vi "F2ToFalseColor.vi"(1 "Intensity":u32[][][][](array[numeric]), 2 "Plane":u32, 3 "Threshold (max)":cluster{"max":u32, "min":u32}) -> (0 "FalseColor":u32[][](array[numeric]))   [LabVIEW 2009]
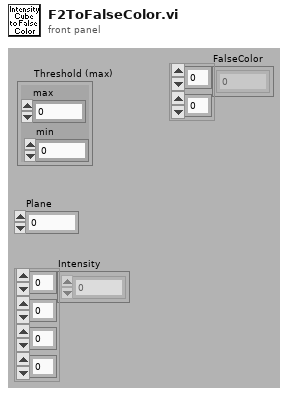
[diagram p1: front panel]
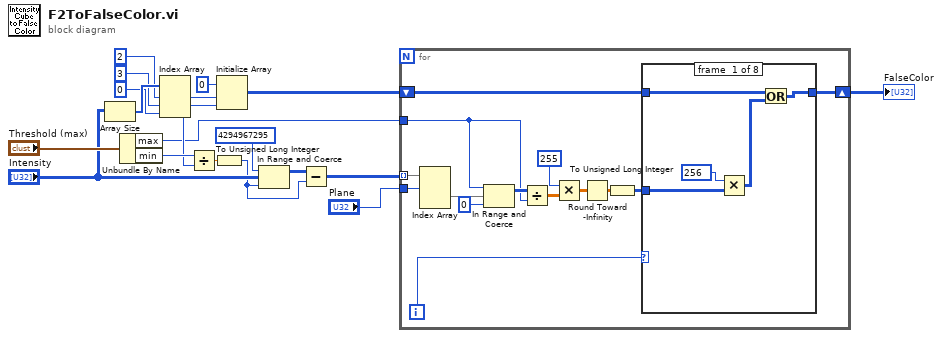
[diagram p0: block diagram]
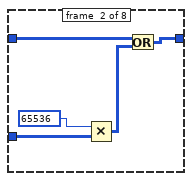
[diagram p2: hidden frame]
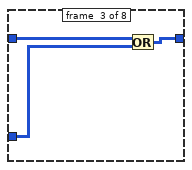
[diagram p3: hidden frame]
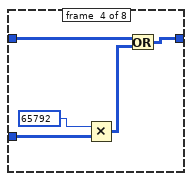
[diagram p4: hidden frame]
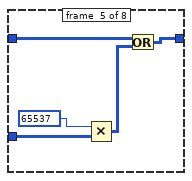
[diagram p5: hidden frame]
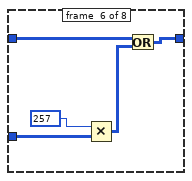
[diagram p6: hidden frame]
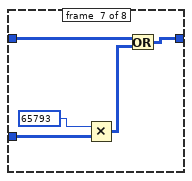
[diagram p7: hidden frame]
diagram:
  n1 = Array Size(array="Intensity") -> (size(s)=w17:i32[])
  n2 = Unbundle By Name("Threshold (max)") -> ("max"=w1:u32, "min"=w9:u32)
  n3 = Index Array(array=w17, index #1=2 ("index"), index #2=3 ("index"), index #3=0 ("index")) -> (element #1=w11:i32, element #2=w10:i32, element #3=w8:i32)
  n4 = Divide(x=w9, y=w8) -> (x/y=w7:dbl)
  n5 = To Unsigned Long Integer(number=w7) -> (unsigned 32bit integer=w4:u32)
  n6 = Initialize Array(u32 0, w11, w10) -> (w14:u32[][])
  n7 = In Range and Coerce(upper limit=u32 4294967295 ("index"), x="Intensity", lower limit=w4) -> (coerced(x)=w5:u32[][][][])  [unwired: 1 out]
  n8 = Subtract(x=w5, y=w4) -> (x-y=w2:u32[][][][])
  n9 = for {
    tunnel: w2 -> [w34] mode=indexing
    tunnel: "Plane" -> [w33]
    shift-right: [w22] -> w20
    shift-left: w14 -> [w23]
    tunnel: w1 -> [w21]
    i -> [w30]
    n10 = Index Array(array=w34, index (dim 0)=w33) -> (element=w32:u32[][])  [unwired: 2 in]
    n11 = In Range and Coerce(upper limit=w21, x=w32, lower limit=u32 0) -> (coerced(x)=w29:u32[][])  [unwired: 1 out]
    n12 = Divide(x=w29, y=w21) -> (x/y=w28:dbl[][])
    n13 = Multiply(x=u32 255 ("Threshold (max)"), y=w28) -> (x*y=w26:dbl[][])
    n14 = Round Toward -Infinity(1:w26) -> (0:w25:dbl[][])
    n15 = To Unsigned Long Integer(number=w25) -> (unsigned 32bit integer=w24:u32[][])
    n16 = case shown="3" w30 {
      tunnel: w24 -> [w39 w44 w45 w52 w57 w62 w67 _]
      tunnel: w23 -> [w36 w41 w47 w49 w54 w59 w64 w68]
      tunnel: [w35 w40 w46 w48 w53 w58 w63 w68] -> w22
      frame #0 {
        n17 = Multiply(x=u32 256 ("Threshold (max)"), y=w39) -> (x*y=w37:u32[][])
        n18 = Or(x=w36, y=w37) -> (x .or. y?=w35:u32[][])
      }
      frame #1 {
        n19 = Multiply(x=u32 65536 ("Threshold (max)"), y=w44) -> (x*y=w42:u32[][])
        n20 = Or(x=w41, y=w42) -> (x .or. y?=w40:u32[][])
      }
      frame #2 {
        n21 = Or(x=w47, y=w45) -> (x .or. y?=w46:u32[][])
      }
      frame #3 {
        n22 = Multiply(x=u32 65792 ("Threshold (max)"), y=w52) -> (x*y=w50:u32[][])
        n23 = Or(x=w49, y=w50) -> (x .or. y?=w48:u32[][])
      }
      frame #4 {
        n24 = Multiply(x=u32 65537 ("Threshold (max)"), y=w57) -> (x*y=w55:u32[][])
        n25 = Or(x=w54, y=w55) -> (x .or. y?=w53:u32[][])
      }
      frame #5 {
        n26 = Multiply(x=u32 257 ("Threshold (max)"), y=w62) -> (x*y=w60:u32[][])
        n27 = Or(x=w59, y=w60) -> (x .or. y?=w58:u32[][])
      }
      frame #6 {
        n28 = Multiply(x=u32 65793 ("Threshold (max)"), y=w67) -> (x*y=w65:u32[][])
        n29 = Or(x=w64, y=w65) -> (x .or. y?=w63:u32[][])
      }
      frame #7 {
      }
    }
  }
  "FalseColor" <- w20
